vi "GT Get Crd Segment Time.vi"(0 "cardNum":i16, 1 "pSegmentNumber":i32, 5 "crd":i16, 7 "segmentIndex":i32, 9 "pSegmentTime":dbl, 11 "error in (no error)":errorcluster caption="错误输入（无错误）", 12 "fifo":i16) -> (3 "pSegmentNumber out":i32, 4 "function return":i16, 10 "pSegmentTime out":dbl, 15 "error out":errorcluster caption="错误输出")   [LabVIEW 2014, in "gts.lvlib"]
doc: "GT_API GT_GetCrdSegmentTime(short cardNum,short crd,long segmentIndex,double *pSegmentTime,long *pSegmentNumber,short fifo);"
uses:
  gts.lvlib
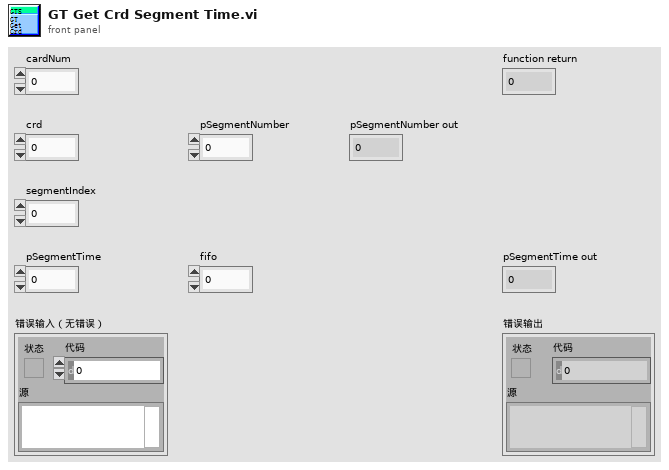
[diagram p1: front panel]
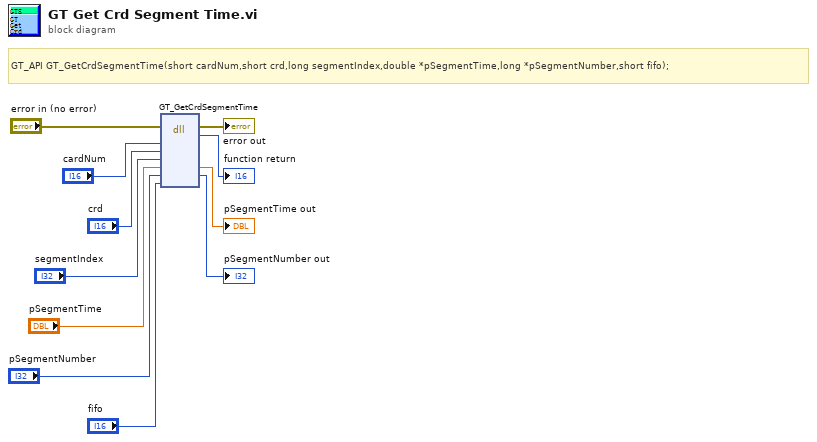
[diagram p0: block diagram]
diagram:
  # "GT_API GT_GetCrdSegmentTime(short cardNum,short crd,long segmentIndex,double *pSegmentTime,long *pSegmentNumber,short fifo);"
  n1 = dll-call lib="PTH2habs D固高科技资料GTS控制卡GTS卡18年上半年资料dllVC32bit\nmulti_cardgts.*" fn="GT_GetCrdSegmentTime"(error in="error in (no error)", "cardNum"="cardNum", "crd"="crd", "segmentIndex"="segmentIndex", "pSegmentTime"="pSegmentTime", "pSegmentNumber"="pSegmentNumber", "fifo"="fifo") -> (error out=→"error out":errorcluster, →"function return":i16, "pSegmentTime"=→"pSegmentTime out":dbl, "pSegmentNumber"=→"pSegmentNumber out":i32)  [unwired: 6 in, 1 out]
